vi "KeyPress.vi"(1 "error in (no error)":errorcluster, 3 "Virtual Key":u8(ring)=9) -> (0 "error out":errorcluster)   [LabVIEW 2013]
doc: "This VI simulates Keyboard events by making calls into the keyb_event function of the Windows User32.dll\n\nInstructions:\n1) Run the program\n2) Press the keys in the order you would like to simulate them\n Example 1: With several applications open, press Alt, Tab, Tab, Tab, Alt\n Example 2: Alt, F, Alt, O, A, B, C\n3) Press the Execute button to watch the code simulate the keyboard events"
uses:
  user32.dll
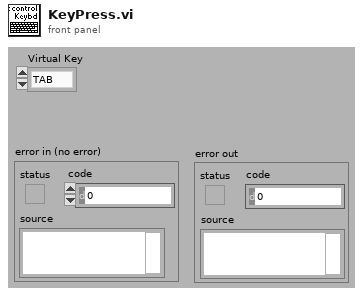
[diagram p1: front panel]
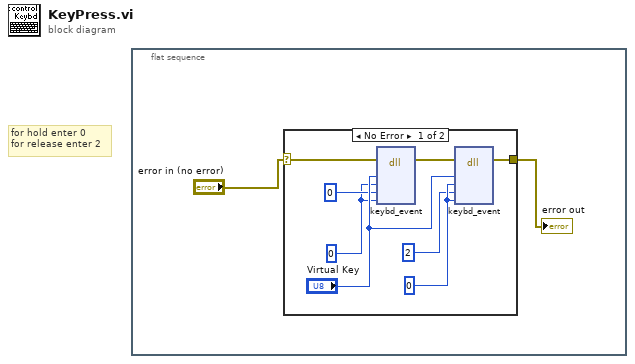
[diagram p0: block diagram]
diagram:
  # "for hold enter 0\nfor release enter 2"
  n1 = flat-sequence {
    frame #0 {
      n2 = case shown="No Error" "error in (no error)" {
        selector: "error in (no error)" -> [w5 w11]
        tunnel: [w9 w11] -> w1
        frame No Error {
          w7 = u32 0 ("dwFlags")
          w3 = u32 0 ("dwFlags")
          n3 = dll-call lib="user32.*" fn="keybd_event"(error in=w5, "bVk"="Virtual Key", "bScan"=w3, "dwFlags"=0 ("HOLD/RELEASE"), "dwExtraInfo"=w3) -> (error out=w10:errorcluster)  [unwired: 7 in, 1 out]
          n4 = dll-call lib="user32.*" fn="keybd_event"(error in=w10, "bVk"="Virtual Key", "bScan"=w7, "dwFlags"=2 ("HOLD/RELEASE 2"), "dwExtraInfo"=w7) -> (error out=w9:errorcluster)  [unwired: 7 in, 1 out]
        }
        frame Error {
        }
      }
      "error out" <- w1
    }
  }
